vi "Read Device Information.vi"(8 "error in (no error)":errorcluster, 11 "VGC in":refnum<class "PL Inficon VGC.lvclass">) -> (0 "error out":errorcluster, 2 "information":T1, 3 "VGC out":refnum<class "PL Inficon VGC.lvclass">)   [LabVIEW 2015, in "PL Inficon VGC.lvclass"]
doc: "Reads device information."
uses:
  PL Inficon VGC.lvclass
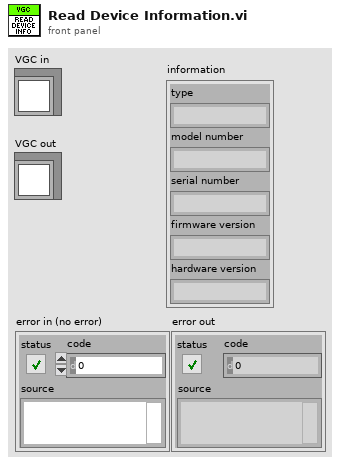
[diagram p1: front panel]
types:
  T1 = cluster{"type":string, "model number":string, "serial number":string, "firmware version":string, "hardware version":string}
  T2 = cluster{"response data[0]":string, "response data[1]":string, "response data[2]":string, "response data[3]":string, "response data[4]":string}
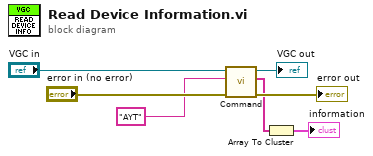
[diagram p0: block diagram]
diagram:
  n1 = call "Command.vi"("error in (no error)"="error in (no error)", "command"="AYT", "VGC in"="VGC in") -> ("error out"=→"error out":errorcluster, "response data"=w2:string[], "VGC out"=→"VGC out":refnum<class "PL Inficon VGC.lvclass">)  [unwired: 6 in]
  n2 = Array To Cluster(array=w2) -> (cluster=→"information":T2)
